vi "Handle Pending Calibration Take Sample.vi"(8 "error in (no error)":errorcluster, 9 "Detections":T1[](array[typedef]), 10 "ARGB Image (duplicate)":T4, 11 "App in":refnum<class "App.lvclass">) -> (0 "error out":errorcluster, 3 "App out":refnum<class "App.lvclass">)   [LabVIEW 2020, in "AR Example.lvlib" / "App.lvclass"]
uses:
  App.lvclass
  App.lvclass/App.ctl
  UI/UI.lvclass
  g_ar_toolkit.image/New Image (ARGB).vi
  g_ar_toolkit.image/Resize (ARGB).vi
  g_ar_toolkit.image/Size (ARGB).vi
  g_ar_toolkit.common/Image Point (Float).ctl
  g_ar_toolkit.common/Square Corners.ctl
  g_ar_toolkit.feature_detection/Apriltag Detector/Detection.ctl
  g_ar_toolkit.image/ARGB Image.ctl
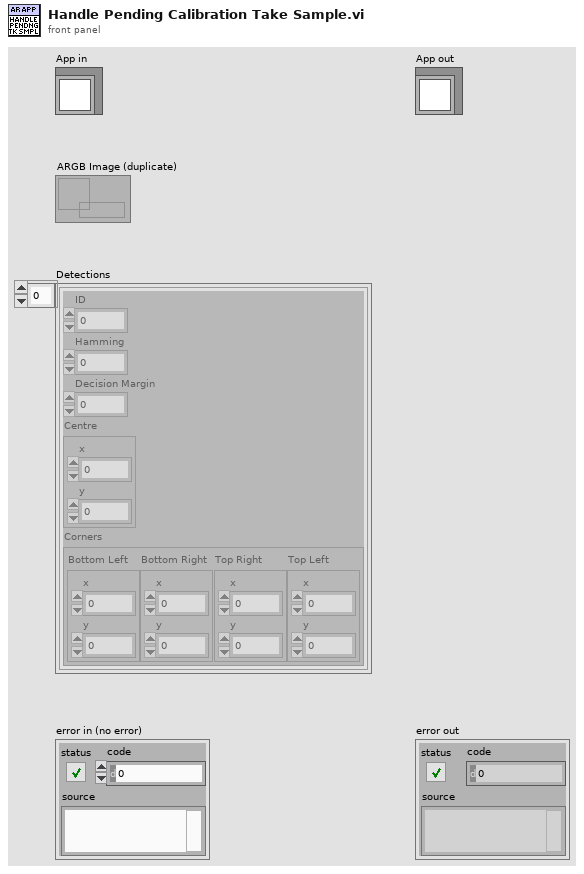
[diagram p1: front panel]
types:
  T1 = typedef "g_ar_toolkit.feature_detection.lvlib/AprilTag Detector.lvclass/Detection.ctl" = cluster{"ID":i32, "Hamming":i32, "Decision Margin":sgl, "Centre":T2, "Corners":T3}
  T2 = typedef "g_ar_toolkit.common.lvlib/Image Point (Float).ctl" = cluster{"x":dbl, "y":dbl}
  T3 = typedef "g_ar_toolkit.common.lvlib/Square Corners.ctl" = cluster{"Bottom Left":T2, "Bottom Right":T2, "Top Right":T2, "Top Left":T2}
  T4 = typedef "g_ar_toolkit.image.lvlib/ARGB Image.ctl" = refnum<data-value>
  T5 = typedef "g_ar_toolkit.common.lvlib/Object Point (Float).ctl" = cluster{"x":dbl, "y":dbl, "z":dbl}
  T6 = typedef "g_ar_toolkit.common.lvlib/Image Size (Integer).ctl" = cluster{"Width":u16, "Height":u16}
  T7 = cluster{"Detections":T1[], "Cal Image":refnum<data-value>}[]
  T8 = cluster{"Detections":T1[], "ARGB  Destination Image (duplicate)":T4}
  T9 = cluster{"Detections":T1[], "ARGB  Destination Image (duplicate)":T4}[]
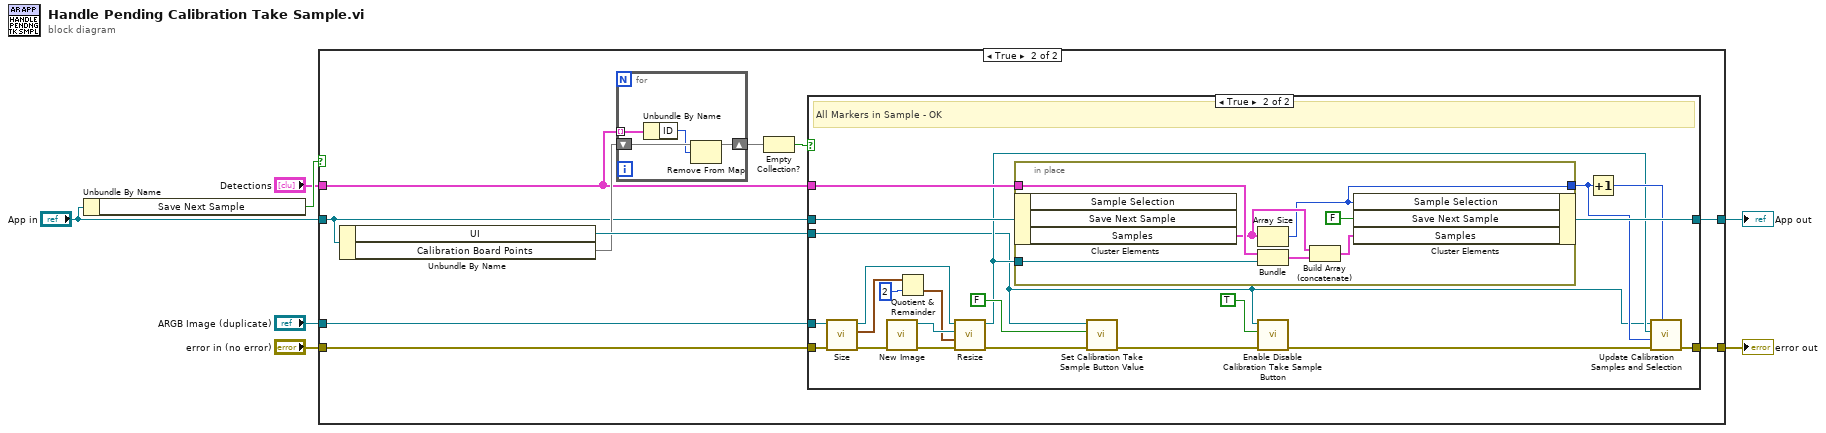
[diagram p0: block diagram]
diagram:
  n1 = Unbundle By Name("App in") -> ("Save Next Sample"=w3:bool)
  n2 = case shown="True" w3 {
    tunnel: "error in (no error)" -> [w9 w18]
    tunnel: [w9 w17] -> w6
    tunnel: "App in" -> [w8 w14]
    tunnel: [w8 w13] -> w7
    tunnel: "ARGB Image (duplicate)" -> [_ w11]
    tunnel: "Detections" -> [_ w10]
    frame False {
    }
    frame True {
      n3 = Unbundle By Name(w14) -> ("UI"=w19:refnum<class "UI.lvclass">, "Calibration Board Points"=w16:map{i32, T5[]})
      n4 = for {
        tunnel: w10 -> [w52] mode=indexing
        shift-right: [w53] -> w15
        shift-left: w16 -> [w54]
        n5 = Unbundle By Name(w52) -> ("ID"=w51:i32)
        n6 = Remove From Map(10:w51, 11:w54) -> (3:w53:map{i32, T5[]})  [unwired: 2 out]
      }
      n7 = Empty Collection?(1:w15) -> (0:w12:bool)
      n8 = case shown="True" w12 {
        tunnel: w19 -> [_ w22]
        tunnel: w18 -> [w20 w43]
        tunnel: [w20 w26] -> w17
        tunnel: w14 -> [w21 w29]
        tunnel: [w21 w28] -> w13
        tunnel: w11 -> [_ w35]
        tunnel: w10 -> [_ w27]
        frame False {
          # "Not All Markers in Sample"
        }
        frame True {
          # "All Markers in Sample - OK"
          n9 = call-poly "Size.vi"("error in (no error)"=w43, "ARGB Image"=w35) -> ("error out"=w36:errorcluster, "Image Size"=w33:T6, "ARGB Image (duplicate)"=w34:T4)  [unwired: 7 in]
          n10 = call-poly "New Image.vi"("error in (no error)"=w36) -> ("error out"=w38:errorcluster, "New ARGB Image"=w37:T4)  [unwired: 9 in]
          n11 = Quotient & Remainder(x=w33, y=u16 2) -> (floor(x/y)=w31:T6)  [unwired: 1 out]
          n12 = call-poly "Resize.vi"("error in (no error)"=w38, "New Image Size"=w31, "ARGB Destination Image"=w37, "ARGB Source Image"=w34) -> ("error out"=w30:errorcluster, "ARGB  Destination Image (duplicate)"=w23:T4)  [unwired: 6 in]
          n13 = in-place {
            in-place-border: w27 -> [w50]
            in-place-border: w23 -> [w49]
            in-place-border: [w44] -> w24
            n14 = in-place-cluster #1(w29) -> ("Samples"=w46:T7)  [unwired: 2 out]
            n15 = Array Size(array=w46) -> (size(s)=w44:i32)
            n16 = Bundle("Detections"=w50, "ARGB  Destination Image (duplicate)"=w49) -> (w48:T8)  [unwired: 1 in]
            n17 = Build Array (concatenate)(w46, w48) -> (w47:T9)
            n18 = in-place-cluster #1("Sample Selection"=w44, "Save Next Sample"=FALSE ("Camera Calibration.Save Next Sample"), "Samples"=w47) -> (w28:refnum<class "App.lvclass">)
          }
          n19 = call-dynamic "Set Calibration Take Sample Button Value.vi"("error in (no error)"=w30, "Value"=FALSE, "UI in"=w22) -> ("error out"=w40:errorcluster)  [unwired: 8 in]
          n20 = call-dynamic "Enable Disable Calibration Take Sample Button.vi"("error in (no error)"=w40, "Enable?"=TRUE, "UI in"=w22) -> ("error out"=w42:errorcluster)  [unwired: 8 in]
          n21 = Increment(x=w24) -> (x+1=w25:i32)
          n22 = call "Update Calibration Samples and Selection.vi"("N-Samples"=w25, "error in (no error)"=w42, "Selection"=w24, "Sample"=w23, "UI in"=w22) -> ("error out"=w26:errorcluster)  [unwired: 6 in]
        }
      }
    }
  }
  "App out" <- w7
  "error out" <- w6
